vi "Raw_BG_correction_.vi"(8 "error in (no error)":errorcluster caption="entrée d'erreur (pas d'erreur)", 9 "raw bg":i32[](array[numeric]), 11 "Control-Client en entrée":refnum<class "Control-Client.lvclass">) -> (0 "error out":errorcluster caption="sortie d'erreur", 2 "Data corrected":dbl[][](array[numeric]), 3 "Control-Client en sortie":refnum<class "Control-Client.lvclass">)   [LabVIEW 2018, in "Control-Client.lvclass"]
uses:
  Control-Client.lvclass
  Control-Client.lvclass/Control-Client.ctl
  dependecies/average-2Darray-SD_double.vi
  Experiments/Experiment.lvclass
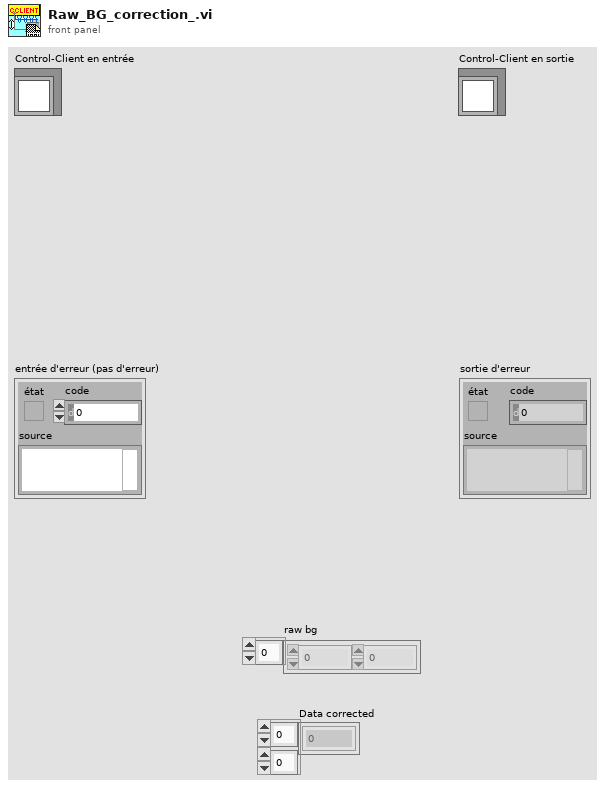
[diagram p1: front panel]
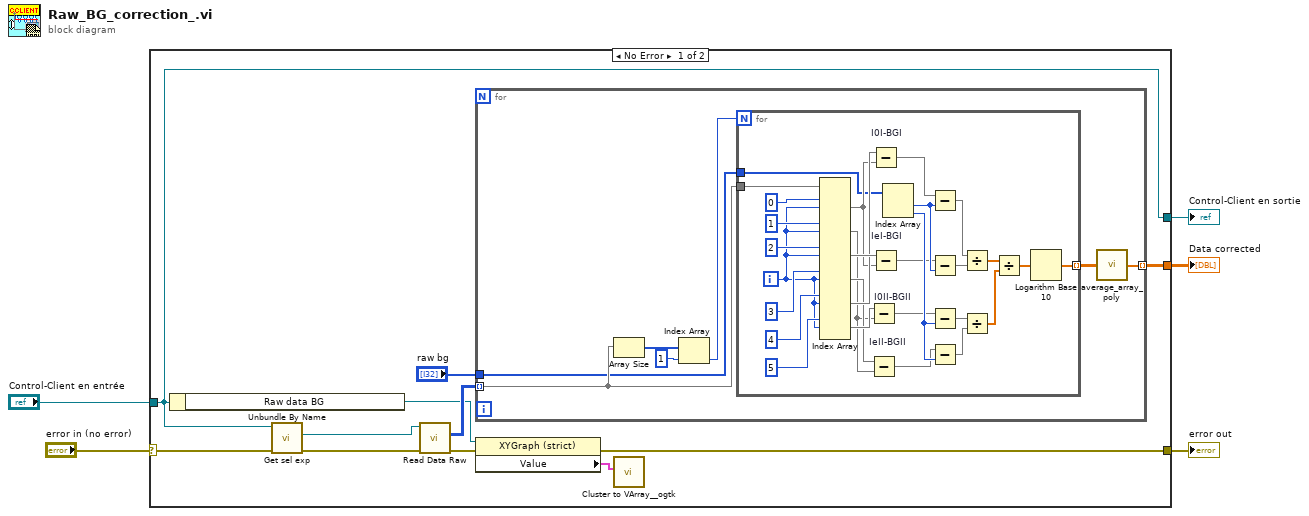
[diagram p0: block diagram]
diagram:
  n1 = case shown="No Error" "error in (no error)" {
    selector: "error in (no error)" -> [w14 w54]
    tunnel: [w15 w54] -> w4
    tunnel: [w10 w53] -> w2
    tunnel: "Control-Client en entrée" -> [w10 w53]
    tunnel: [w16 _] -> w1
    frame No Error {
      n2 = Unbundle By Name(w10) -> ("Raw data BG"=w8:refnum<vi>)
      n3 = call "Get sel exp.vi"("error in (no error)"=w14, "Control-Client in"=w10) -> ("error out"=w13:errorcluster, "Sel experiment"=w11:refnum<class "Experiment.lvclass">)  [unwired: 7 in, 1 out]
      n4 = call-dynamic "Read Data Raw.vi"("error in (no error)"=w13, "Experiment in"=w11) -> ("error out"=w7:errorcluster, "Data Raw"=w12:i32[][][][])  [unwired: 7 in, 1 out]
      n5 = for {
        tunnel: w12 -> [w20] mode=indexing
        tunnel: [w18] -> w16 mode=indexing
        tunnel: "raw bg" -> [w17]
        n6 = Array Size(array=w20) -> (size(s)=w23:i32[])
        n7 = Index Array(array=w23, index=1) -> (element=w21:i32)
        n8 = for {
          N: w21 -> [_]
          tunnel: w20 -> [w52]
          tunnel: [w35] -> w19 mode=indexing
          tunnel: w17 -> [w24]
          i -> [w45]
          n9 = Index Array(array=w52, index (dim 0) #1=0 ("disabled index (page)"), index (dim 1) #1=w45, index (dim 0) #2=1 ("index (page)"), index (dim 1) #2=w45, index (dim 0) #3=2 ("index (page)"), index (dim 1) #3=w45, index (dim 0) #4=3 ("index (page)"), index (dim 1) #4=w45, index (dim 0) #5=4 ("index (page)"), index (dim 1) #5=w45, index (dim 0) #6=5 ("index (page)"), index (dim 1) #6=w45) -> (element #1=w42:i32[], element #2=w39:i32[], element #3=w44:i32[], element #4=w40:i32[], element #5=w43:i32[], element #6=w41:i32[])  [unwired: 6 in]
          n10 = Subtract "I0II-BGII"(x=w41, y=w39) -> (x-y=w25:i32[])
          n11 = Subtract "IeII-BGII"(x=w40, y=w39) -> (x-y=w26:i32[])
          n12 = Subtract "I0I-BGI"(x=w43, y=w42) -> (x-y=w27:i32[])
          n13 = Subtract "IeI-BGI"(x=w44, y=w42) -> (x-y=w28:i32[])
          n14 = Index Array(array=w24) -> (element #1=w30:i32, element #2=w29:i32)  [unwired: 2 in]
          n15 = Subtract(x=w27, y=w30) -> (x-y=w34:i32[])
          n16 = Subtract(x=w28, y=w30) -> (x-y=w33:i32[])
          n17 = Subtract(x=w25, y=w29) -> (x-y=w32:i32[])
          n18 = Subtract(x=w26, y=w29) -> (x-y=w31:i32[])
          n19 = Divide(x=w34, y=w33) -> (x/y=w38:dbl[])
          n20 = Divide(x=w32, y=w31) -> (x/y=w37:dbl[])
          n21 = Divide(x=w38, y=w37) -> (x/y=w36:dbl[])
          n22 = Logarithm Base 10(1:w36) -> (0:w35:dbl[])
        }
        n23 = call-poly "average_array_poly.vi"("2D array"=w19) -> ("out array"=w18:dbl[])
      }
      n24 = property class="XYGraph (strict)"(reference=w8, error in=w7) -> (error out=w15:errorcluster, "Value"=w6:cluster{dbl[], dbl[]}[])  [unwired: 1 out]
      n25 = call <userlib>:"Cluster to VArray__ogtk.vi"("Cluster"=w6) -> ()  [unwired: 9 in, 2 out]
    }
    frame Error {
    }
  }
  "error out" <- w4
  "Control-Client en sortie" <- w2
  "Data corrected" <- w1
